vi "MPM_Get_Trigger_Input_Mode.vi"(8 "error in (no error)":errorcluster, 11 ".NET Reference in":refnum<k24>) -> (0 "error out":errorcluster, 2 "mode":i32(ring) items=["Internal", "Extarnal"], 3 "Reference out":refnum<k24>)   [LabVIEW 2017]
uses:
  D:/test/FULLband-sts/Fullband_Sample/DLL/InstrumentDLL.dll
  DLL/InstrumentDLL.dll
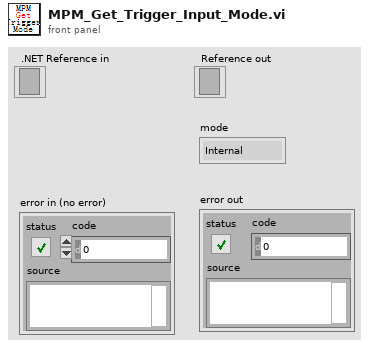
[diagram p1: front panel]
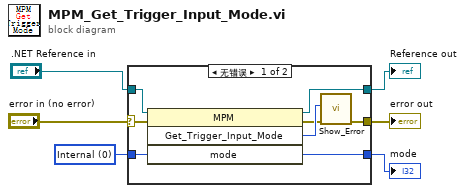
[diagram p0: block diagram]
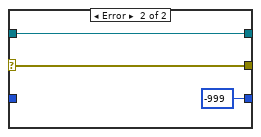
[diagram p2: hidden frame]
diagram:
  w3 = 0 items=["Internal", "Extarnal"] ("mode")
  n1 = case shown="无错误" "error in (no error)" {
    selector: "error in (no error)" -> [w7 w17]
    tunnel: [w14 -999 ("mode")] -> w6
    tunnel: ".NET Reference in" -> [w13 w16]
    tunnel: [w12 w16] -> w4
    tunnel: w3 -> [w11 _]
    tunnel: [w8 w17] -> w2
    frame No Error {
      n2 = invoke class="MPM" method="Get_Trigger_Input_Mode"(reference=w13, error in=w7, "mode"=w11) -> (reference out=w12:refnum<k24>, error out=w9:errorcluster, "Get_Trigger_Input_Mode"=w10:i32, "mode"=w14:i32)  [unwired: 1 in]
      n3 = call "Show_Error.vi"("error in (no error)"=w9, "Error"=w10) -> ("error out"=w8:errorcluster)  [unwired: 9 in]
    }
    frame Error {
    }
  }
  "Reference out" <- w4
  "error out" <- w2
  "mode" <- w6
